vi "Checkbox of Multicolumn.vi"(8 "error in (no error)":errorcluster) -> (0 "error out":errorcluster)   [LabVIEW 2014]
uses:
  <vilib>/Utility/miscctls.llb/LVPointTypeDef.ctl
panel:
  out "選擇Index":i32[](array[numeric])
  out "選擇名稱":string[][](array[string])
  in  "Stop":bool
  in  "All":bool
  in  "File Listbox":i32(listbox)=2 caption="請選測試名稱"
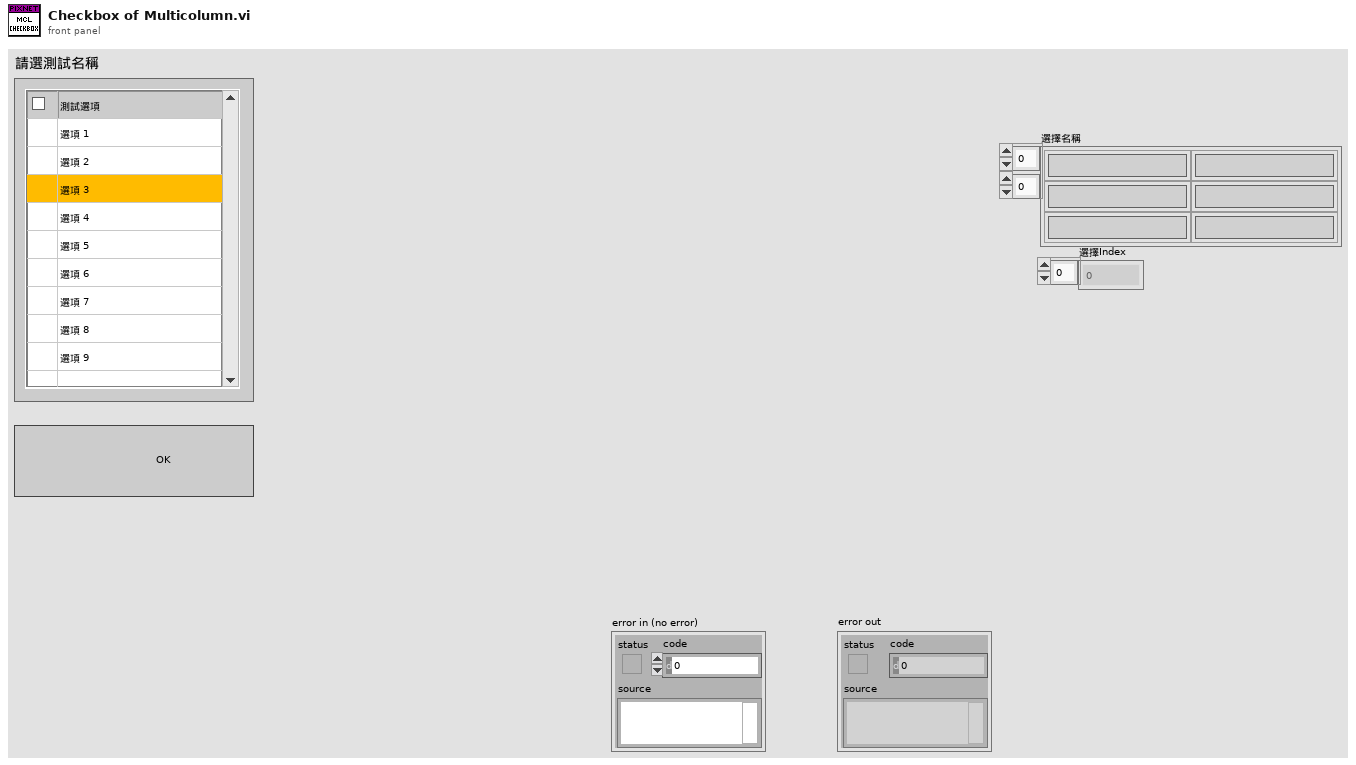
[diagram p1: front panel]
types:
  T1 = typedef "LVPointTypeDef.ctl" = cluster{"Horizontal":i16, "Vertical":i16}
  T2 = typedef "LVPoint32TypeDef.ctl" = cluster{"Horizontal":i32, "Vertical":i32}
  T3 = typedef "LVRowAndColumnTypeDef.ctl" = cluster{"Row":i32, "Column":i32}
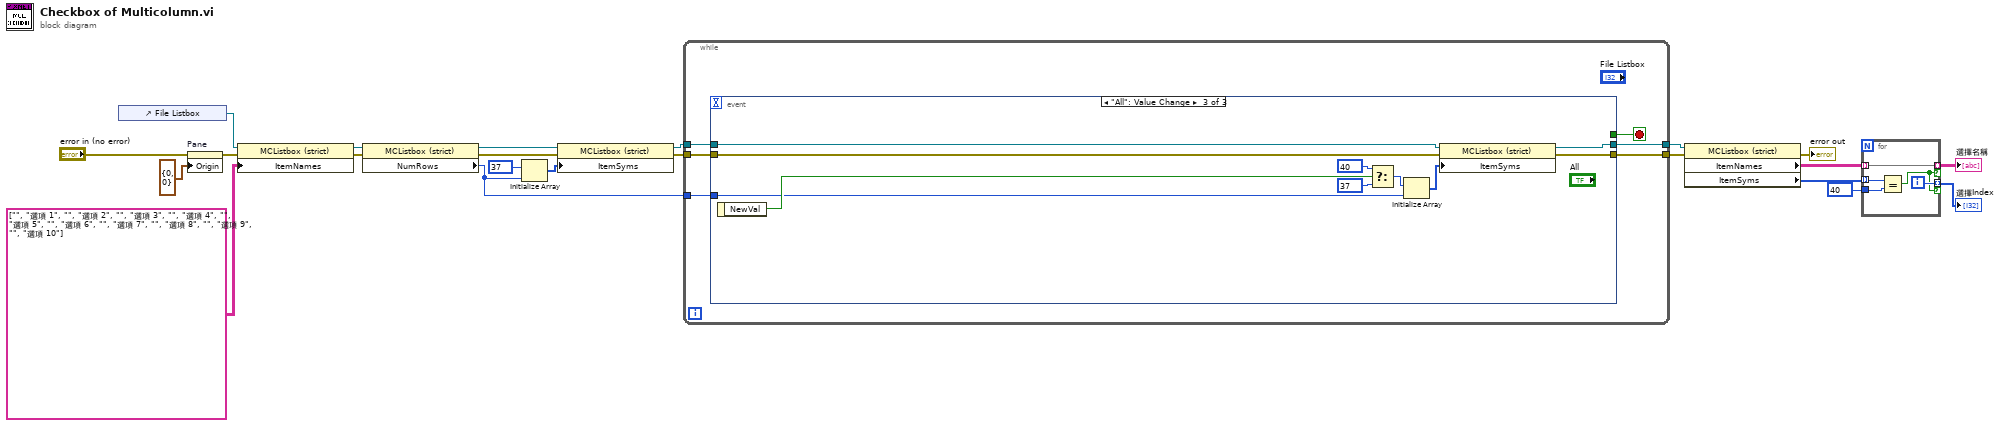
[diagram p0: block diagram]
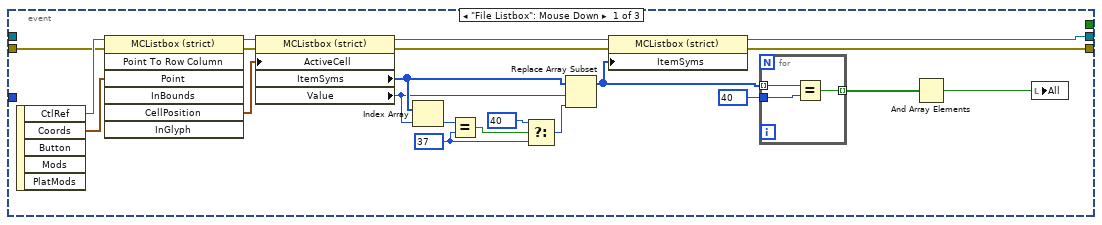
[diagram p2: hidden frame]
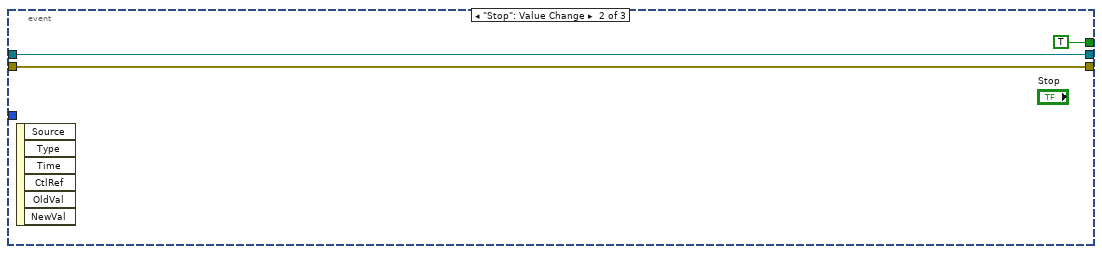
[diagram p3: hidden frame]
diagram:
  n1 = control-ref of="File Listbox"() -> (w16:refnum<vi>)
  n2 = property on="Pane" class="Pane"(error in="error in (no error)", "Origin"=T1 {"Horizontal"=0, "Vertical"=0}) -> (error out=w2:errorcluster)  [unwired: 1 in, 1 out]
  n3 = property on="Property Node" class="MCListbox (strict)"(reference=w16, error in=w2, "ItemNames"=string[][] [["", "選項 1"], ["", "選項 2"], ["", "選項 3"], ["", "選項 4"], ["", "選項 5"], ["", "選項 6"], ["", "選項 7"], ["", "選項 8"], ["", "選項 9"], ["", "選項 10"]]) -> (reference out=w17:refnum<vi>, error out=w18:errorcluster)
  n4 = property on="Property Node" class="MCListbox (strict)"(reference=w17, error in=w18) -> (reference out=w21:refnum<vi>, error out=w20:errorcluster, "NumRows"=w12:u32)
  n5 = Initialize Array(37, w12) -> (w15:i32[])
  n6 = property on="Property Node" class="MCListbox (strict)"(reference=w21, error in=w20, "ItemSyms"=w15) -> (reference out=w22:refnum<vi>, error out=w13:errorcluster)
  n7 = while {
    tunnel: w12 -> [w25]
    tunnel: w22 -> [w24]
    tunnel: w13 -> [w28]
    tunnel: [w27] -> w10
    tunnel: [w23] -> w11
    stop <- w26 stop-if-true
    n8 = event shown="[2] \"All\": Value Change" {
      selector: _ -> [_ _ _]
      dyn-events: _ -> [_ _ _]
      timeout: _ -> [_ _ _]
      tunnel: w28 -> [w45 w55 w58]
      tunnel: [w44 w55 w57] -> w27
      tunnel: [_ TRUE ("NewVal") _] -> w26
      tunnel: w25 -> [_ _ w61]
      tunnel: w24 -> [_ w53 w59]
      tunnel: [w42 w53 w56] -> w23
      event "File Listbox": Mouse Down {
        w35 = 37
        n9 = event-data() -> ("CtlRef"=w49:refnum<vi>, "Coords"=w48:T2)  [unwired: 1 in, 3 out]
        n10 = invoke class="MCListbox (strict)" method="Point To Row Column"(reference=w49, error in=w45, "Point"=w48) -> (reference out=w47:refnum<vi>, error out=w46:errorcluster, "CellPosition"=w43:T3)  [unwired: 4 in, 4 out]
        n11 = property class="MCListbox (strict)"(reference=w47, error in=w46, "ActiveCell"=w43) -> (reference out=w36:refnum<vi>, error out=w32:errorcluster, "ItemSyms"=w30:i32[], "Value"=w29:i32)
        n12 = Index Array(array=w30, index=w29) -> (element=w33:i32)
        n13 = Equal?(x=w33, y=w35) -> (x = y?=w38:bool)
        n14 = Select(t=40, s=w38, f=w35) -> (s? t:f=w37:i32)
        n15 = Replace Array Subset(array=w30, new element=w37, index=w29) -> (w31:i32[])
        n16 = property class="MCListbox (strict)"(reference=w36, error in=w32, "ItemSyms"=w31) -> (reference out=w42:refnum<vi>, error out=w44:errorcluster)
        n17 = for {
          tunnel: w31 -> [w52] mode=indexing
          tunnel: 40 -> [w51]
          tunnel: [w50] -> w40 mode=indexing
          n18 = Equal?(x=w52, y=w51) -> (x = y?=w50:bool)
        }
        n19 = And Array Elements(Boolean array=w40) -> (logical AND=w39:bool)
        n20 = local write "All"(w39) -> ()
      }
      event "Stop": Value Change {
        n21 = event-data() -> ()  [unwired: 1 in, 6 out]
      }
      event "All": Value Change {
        n22 = event-data() -> ("NewVal"=w65:bool)  [unwired: 1 in]
        n23 = Select(t=40, s=w65, f=37) -> (s? t:f=w62:i32)
        n24 = Initialize Array(w62, w61) -> (w60:i32[])
        n25 = property on="Property Node" class="MCListbox (strict)"(reference=w59, error in=w58, "ItemSyms"=w60) -> (reference out=w56:refnum<vi>, error out=w57:errorcluster)
      }
    }
  }
  n26 = property on="Property Node" class="MCListbox (strict)"(reference=w11, error in=w10) -> (error out=→"error out":errorcluster, "ItemNames"=w7:string[][], "ItemSyms"=w8:i32[])  [unwired: 1 out]
  n27 = for {
    tunnel: w8 -> [w70] mode=indexing
    tunnel: 40 -> [w69]
    tunnel: [w68] -> w6 mode=indexing if=w66
    tunnel: w7 -> [w68] mode=indexing
    tunnel: [w67] -> w4 mode=indexing if=w66
    i -> [w67]
    n28 = Equal?(x=w70, y=w69) -> (x = y?=w66:bool)
  }
  "選擇名稱" <- w6
  "選擇Index" <- w4
